vi "Configure parameter.vi"(5 "Board parameter? (F)":bool, 6 "String value":string, 7 "All Channels (F)":bool, 8 "error in (no error)":errorcluster, 9 "Parameter name":string, 10 "Channel (0)":u8, 11 "BoardHandle":T1) -> (0 "error out":errorcluster, 3 "BoardHandle out":T1)   [LabVIEW 2020, in "CAEN PSM.lvlib"]
doc: "This function allows configuring a parameter indicated in the input (both of board and channel). The value to be set is in string format."
uses:
  CAEN PSM.lvlib
  BoardHandle.ctl
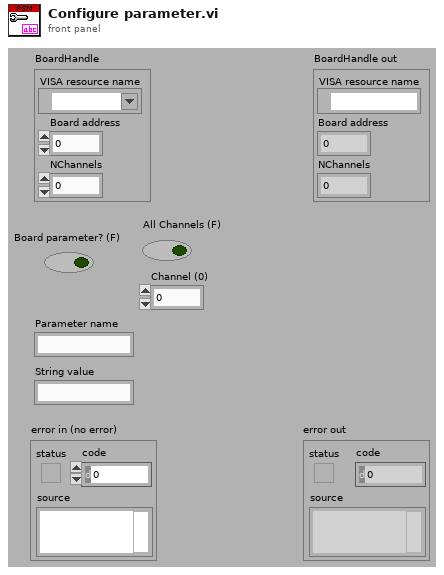
[diagram p1: front panel]
types:
  T1 = typedef "CAEN PSM.lvlib/BoardHandle.ctl" = cluster{"VISA resource name":refnum<visa-resource-name>, "Board address":i8, "NChannels":u8}
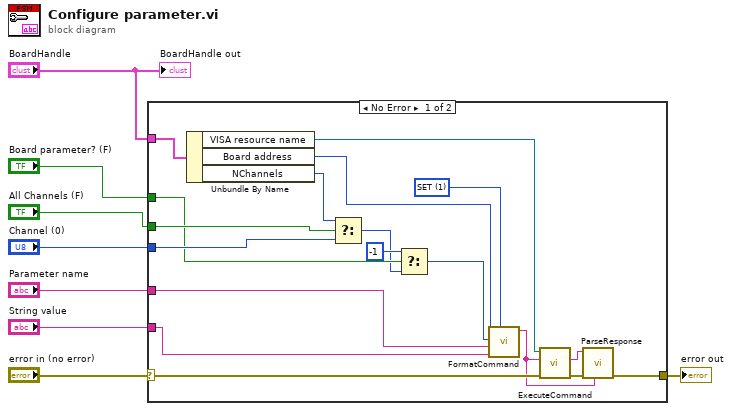
[diagram p0: block diagram]
diagram:
  n1 = case shown="No Error" "error in (no error)" {
    selector: "error in (no error)" -> [w16 w27]
    tunnel: "All Channels (F)" -> [w24 _]
    tunnel: "Channel (0)" -> [w22 _]
    tunnel: [w19 w27] -> w5
    tunnel: "BoardHandle" -> [w17 _]
    tunnel: "String value" -> [w15 _]
    tunnel: "Parameter name" -> [w14 _]
    tunnel: "Board parameter? (F)" -> [w13 _]
    frame No Error {
      w25 = u8 1 items=["MON", "SET"] ("CMD")
      n2 = Unbundle By Name(w17) -> ("VISA resource name"=w21:refnum<visa-resource-name>, "Board address"=w26:i8, "NChannels"=w23:u8)
      n3 = Select(t=w23, s=w24, f=w22) -> (s? t:f=w10:u8)
      n4 = Select(t=i8 -1, s=w13, f=w10) -> (s? t:f=w11:u8)
      n5 = call "FormatCommand.vi"("CMD (MON)"=w25, "VAL"=w15, "PAR"=w14, "CH"=w11, "BD (0)"=w26) -> ("cmd"=w9:string)  [unwired: 6 in]
      n6 = call "ExecuteCommand.vi"("error in (no error)"=w16, "Command"=w9, "VISA resource name"=w21) -> ("error out"=w20:errorcluster, "Response"=w18:string)  [unwired: 6 in, 1 out]
      n7 = call "ParseResponse.vi"("Command"=w9, "error in (no error)"=w20, "Response"=w18) -> ("error out"=w19:errorcluster)  [unwired: 5 in, 3 out]
    }
    frame Error {
    }
  }
  "error out" <- w5
  "BoardHandle out" <- "BoardHandle"
